vi "sendServerNotification.vi"(8 "error in (no error)":errorcluster, 10 "connectionStatus":bool, 11 "TcpServerBase in":refnum<class "TcpServerBase.lvclass">) -> (0 "error out":errorcluster, 3 "TcpServerBase out":refnum<class "TcpServerBase.lvclass">)   [LabVIEW 2018, in "TcpServerBase.lvclass"]
doc: "Send a notification when TCP Client connects or disconnects.\n\nNOTE: put the VI in preallocated reentrant clone execution."
uses:
  TcpServerBase.lvclass
  TcpServerBase.lvclass/TcpServerBase.ctl
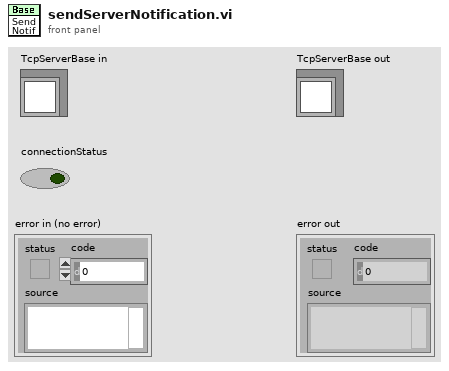
[diagram p1: front panel]
types:
  T1 = cluster{"connectionStatus":bool, "errorSource":string}
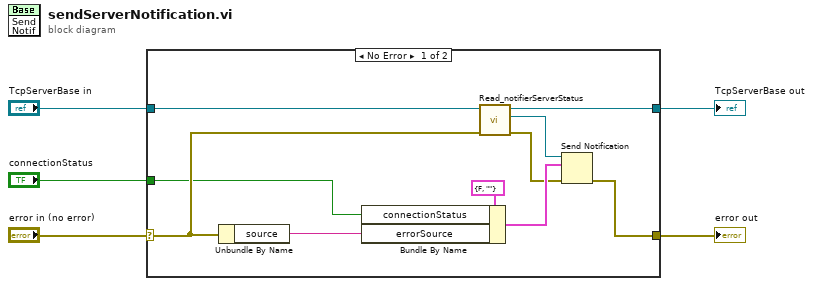
[diagram p0: block diagram]
diagram:
  n1 = case shown="No Error" "error in (no error)" {
    selector: "error in (no error)" -> [w12 w17]
    tunnel: [w6 w17] -> w4
    tunnel: [w7 w16] -> w2
    tunnel: "TcpServerBase in" -> [w15 w16]
    tunnel: "connectionStatus" -> [w10 _]
    frame No Error {
      n2 = Unbundle By Name(w12) -> ("source"=w11:string)
      n3 = Bundle By Name(cluster=T1 {"connectionStatus"=FALSE, "errorSource"=""} ("notification"), "connectionStatus"=w10, "errorSource"=w11) -> (w9:T1)
      n4 = call "Read_notifierServerStatus.vi"("error in (no error)"=w12, "TcpServerBase in"=w15) -> ("error out"=w8:errorcluster, "notifierServerStatus"=w14:refnum<notifier>, "TcpServerBase out"=w7:refnum<class "TcpServerBase.lvclass">)  [unwired: 7 in]
      n5 = Send Notification(notification=w9, notifier=w14, error in (no error)=w8) -> (error out=w6:errorcluster)  [unwired: 1 out]
    }
    frame Error {
    }
  }
  "error out" <- w4
  "TcpServerBase out" <- w2
